vi "timestamp_conversion.vi"(7 "error in (no error)":errorcluster, 10 "Time Stamp":timestamp) -> (0 "error out":errorcluster, 3 "Integer Time":i64)   [LabVIEW 2012]
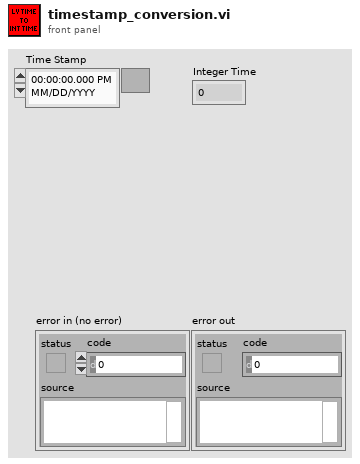
[diagram p1: front panel]
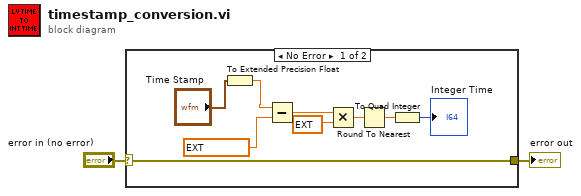
[diagram p0: block diagram]
diagram:
  n1 = case shown="No Error" "error in (no error)" {
    selector: "error in (no error)" -> [w11 w12]
    tunnel: [w11 w12] -> w1
    frame No Error {
      n2 = To Extended Precision Float(1:"Time Stamp") -> (0:w3:ext)
      n3 = Subtract(x=w3, y=ext 2082844800.0) -> (x-y=w9:ext)
      n4 = Multiply(x=w9, y=ext 1000.0) -> (x*y=w6:ext)
      n5 = Round To Nearest(number=w6) -> (nearest integer value=w5:ext)
      n6 = To Quad Integer(1:w5) -> (0:→"Integer Time":i64)
    }
    frame Error {
    }
  }
  "error out" <- w1
